vi "CustomError.vi"(8 "Error In":errorcluster, 11 "Error code":i32) -> (0 "Error Out":errorcluster)   [LabVIEW 2019, in "Tools.lvlib"]
doc: "This FGV outputs an error from <b>Custom errors.csv</b> or <b>TMOS_Errors.csv</b> file basing on <b>Error code</b> input."
uses:
  Tools.lvlib
  TMOS/Path/TMOS.Path.Type.ctl
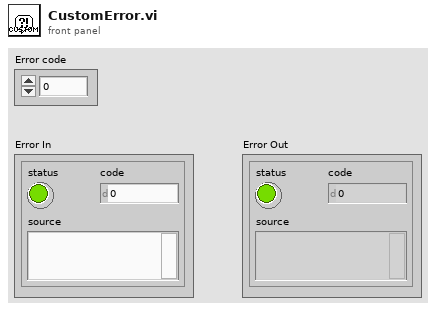
[diagram p1: front panel]
types:
  T1 = typedef "TMOS.Path.Type.ctl" = enum16{"TMOS Configuration file", "Resources directory", "Root directory", "Settings directory", "Verification file", "Users file", "Logs directory", "Drivers directory"}
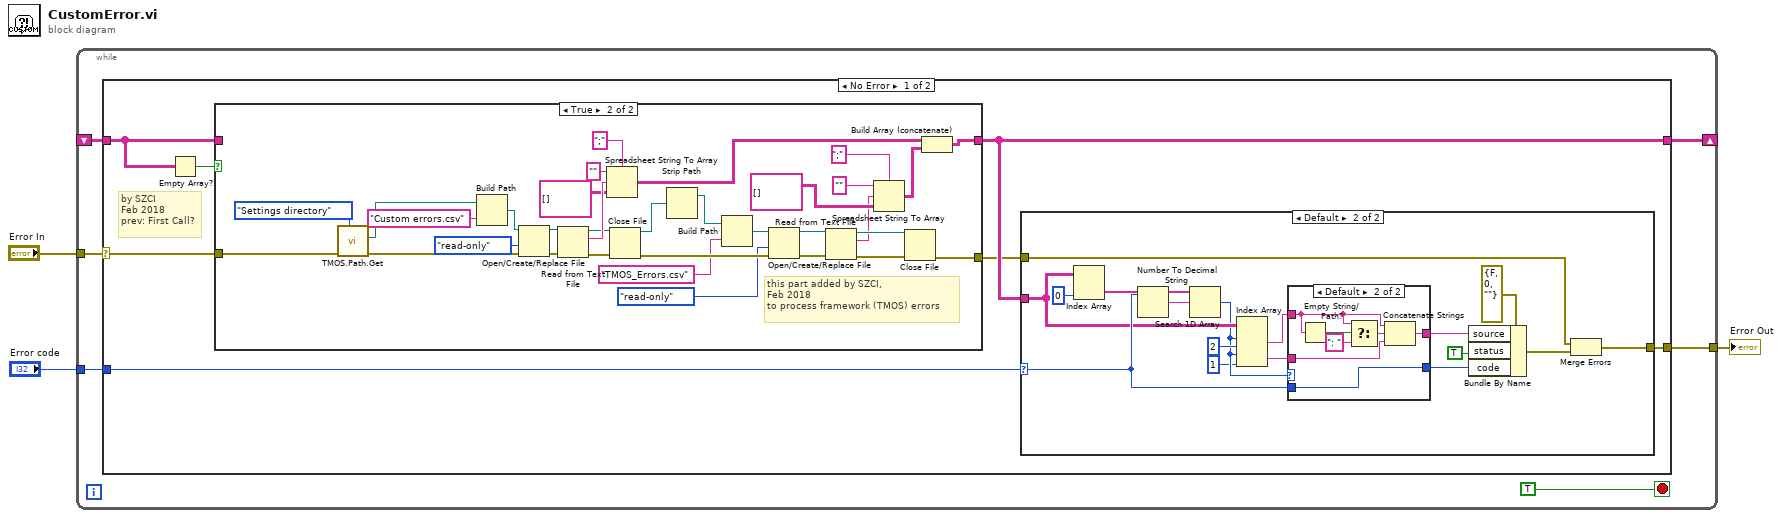
[diagram p0: block diagram]
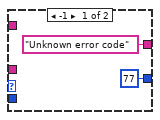
[diagram p4: hidden frame]
diagram:
  n1 = while {
    tunnel: [w8] -> w3
    tunnel: "Error In" -> [w7]
    tunnel: "Error code" -> [w6]
    shift-right: [w4] -> _
    shift-left: _ -> [w5]
    stop <- TRUE stop-if-true
    n2 = case shown="No Error" w7 {
      selector: w7 -> [w12 w80]
      tunnel: w6 -> [w15 _]
      tunnel: [w16 w80] -> w8
      tunnel: w5 -> [w11 w79]
      tunnel: [w14 w79] -> w4
      frame No Error {
        # "by SZCI\nFeb 2018\nprev: First Call?"
        n3 = Empty Array?(array=w11) -> (empty?=w10:bool)
        n4 = case shown="True" w10 {
          tunnel: [w18 w25] -> w14
          tunnel: w11 -> [w18 _]
          tunnel: [w17 w30] -> w13
          tunnel: w12 -> [w17 w40]
          frame False {
          }
          frame True {
            # "this part added by SZCI,\nFeb 2018\nto process framework (TMOS) errors"
            n5 = call "TMOS.Path.Get.vi"("type"=TMOS.Path.Type."Settings directory", "error in"=w40) -> ("error out"=w39:errorcluster, "path"=w41:path)  [unwired: 7 in, 1 out]
            n6 = Build Path(base path=w41, name or relative path="Custom errors.csv") -> (appended path=w51:path)
            n7 = Open/Create/Replace File(file path (use dialog)=w51, error in=w39, access (0:read/write)=enum16{"read/write", "read-only", "write-only"}."read-only") -> (refnum out=w46:refnum<file>, error out=w44:errorcluster)  [unwired: 3 in, 1 out]
            n8 = Read from Text File(file (use dialog)=w46, error in=w44) -> (refnum out=w43:refnum<file>, text=w48:string, error out=w42:errorcluster)  [unwired: 2 in, 1 out]
            n9 = Spreadsheet String To Array(delimiter (Tab)=";", format string="", spreadsheet string=w48, array type (2D Dbl)=string[][] []) -> (array=w38:string[][])
            n10 = Close File(refnum=w43, error in=w42) -> (path=w22:path, error out=w33:errorcluster)
            n11 = Strip Path(path=w22) -> (stripped path=w20:path)  [unwired: 1 out]
            n12 = Build Path(base path=w20, name or relative path="TMOS_Errors.csv") -> (appended path=w21:path)
            n13 = Open/Create/Replace File(file path (use dialog)=w21, error in=w33, access (0:read/write)=enum16{"read/write", "read-only", "write-only"}."read-only") -> (refnum out=w34:refnum<file>, error out=w32:errorcluster)  [unwired: 3 in, 1 out]
            n14 = Read from Text File(file (use dialog)=w34, error in=w32) -> (refnum out=w35:refnum<file>, text=w26:string, error out=w31:errorcluster)  [unwired: 2 in, 1 out]
            n15 = Spreadsheet String To Array(delimiter (Tab)=";", format string="", spreadsheet string=w26, array type (2D Dbl)=string[][] []) -> (array=w24:string[][])
            n16 = Close File(refnum=w35, error in=w31) -> (error out=w30:errorcluster)  [unwired: 1 out]
            n17 = Build Array (concatenate)(w38, w24) -> (w25:string[][])
          }
        }
        n18 = case shown="Default" w15 {
          selector: w15 -> [_ w65]
          tunnel: [w52 w55] -> w16
          tunnel: w13 -> [w52 w54]
          tunnel: w14 -> [_ w64]
          frame 0 {
          }
          frame Default {
            n19 = Index Array(array=w64, index (col)=0 ("disabled index (col)")) -> (element=w69:string[])  [unwired: 1 in]
            n20 = Number To Decimal String(number=w65) -> (decimal integer string=w68:string)  [unwired: 1 in]
            n21 = Search 1D Array(1D array=w69, element=w68) -> (index of element=w62:i32)  [unwired: 1 in]
            n22 = Index Array(array=w64, index (row) #1=w62, index (col) #1=2 ("disabled index (col)"), index (row) #2=w62, index (col) #2=1 ("disabled index (col)")) -> (element #1=w66:string, element #2=w60:string)
            n23 = case shown="Default" w62 {
              tunnel: [77 ("error code (0)") w78] -> w58
              tunnel: w65 -> [_ w78]
              tunnel: w66 -> [_ w72]
              tunnel: ["Unknown error code" ("error message (\"\")") w77] -> w56
              tunnel: w60 -> [_ w76]
              frame -1 {
              }
              frame Default {
                n24 = Empty String/Path?(string/path=w72) -> (empty?=w74:bool)
                n25 = Select(t=w72, s=w74, f=": " ("string")) -> (s? t:f=w73:string)
                n26 = Concatenate Strings(w72, w73, w76) -> (w77:string)
              }
            }
            n27 = Bundle By Name(cluster=errorcluster {"status"=FALSE, "code"=0, "source"=""} ("error out"), "source"=w56, "status"=TRUE, "code"=w58) -> (w59:errorcluster)
            n28 = Merge Errors(w54, w59) -> (w55:errorcluster)
          }
        }
      }
      frame Error {
      }
    }
  }
  "Error Out" <- w3
